vi "Apply Package Name.vi"(8 "error in":errorcluster, 10 "Package Name":string, 11 "gRPC Message Metadata in":T1[](array[typedef])) -> (0 "error out":errorcluster, 3 "gRPC Message Metadata":T1[](array[typedef]))   [LabVIEW 2019, in "grpc-lvsupport.lvlib"]
uses:
  grpc-lvsupport.lvlib
  Message Metadata.ctl
  Message Element Metadata.ctl
  Message Element Type.ctl
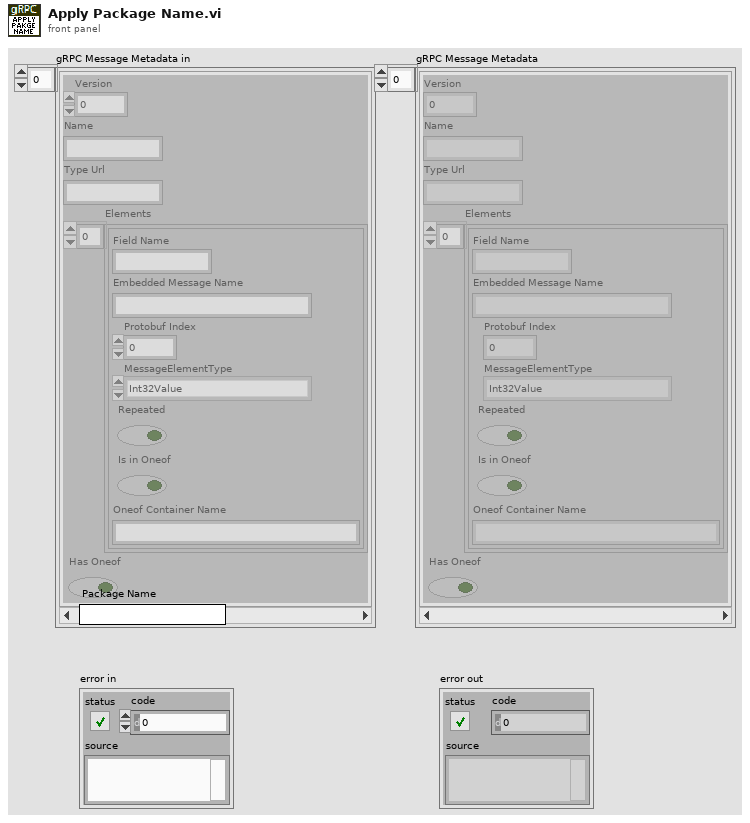
[diagram p1: front panel]
types:
  T1 = typedef "grpc-lvsupport.lvlib/Message Metadata.ctl" = cluster{"Version":i32, "Name":string, "Type Url":string, "Elements":T2[], "Has Oneof":bool}
  T2 = typedef "grpc-lvsupport.lvlib/Message Element Metadata.ctl" = cluster{"Field Name":string, "Embedded Message Name":string, "Protobuf Index":i32, "MessageElementType":T3, "Repeated":bool, "Is in Oneof":bool, "Oneof Container Name":string}
  T3 = typedef "grpc-lvsupport.lvlib/Message Element Type.ctl" = enum32{"Int32Value", "FloatValue", "DoubleValue", "BoolValue", "StringValue", "MessageValue", "Int64Value", "UInt32Value", "UInt64Value", "EnumValue", "Bytes", "Fixed64", "Fixed32", "SFixed64", "SFixed32", "SInt64", "SInt32"}
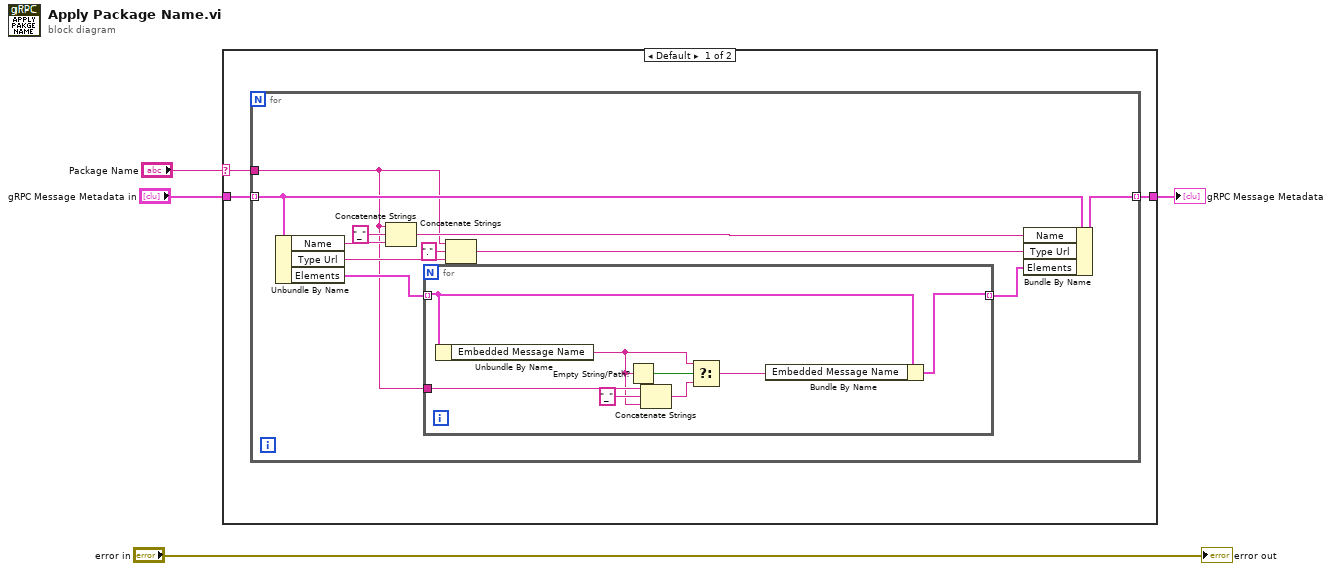
[diagram p0: block diagram]
diagram:
  n1 = case shown="Default" "Package Name" {
    selector: "Package Name" -> [w5 _]
    tunnel: "gRPC Message Metadata in" -> [w7 w27]
    tunnel: [w6 w27] -> w2
    frame Default {
      n2 = for {
        tunnel: w7 -> [w13] mode=indexing
        tunnel: w5 -> [w8]
        tunnel: [w10] -> w6 mode=indexing
        n3 = Unbundle By Name(w13) -> ("Name"=w17:string, "Type Url"=w14:string, "Elements"=w18:T2[])
        n4 = Concatenate Strings(w8, "_" ("string"), w17) -> (w12:string)
        n5 = for {
          tunnel: w18 -> [w23] mode=indexing
          tunnel: [w21] -> w9 mode=indexing
          tunnel: w8 -> [w20]
          n6 = Unbundle By Name(w23) -> ("Embedded Message Name"=w19:string)
          n7 = Empty String/Path?(string/path=w19) -> (empty?=w24:bool)
          n8 = Concatenate Strings(w20, "_" ("string"), w19) -> (w25:string)
          n9 = Select(t=w19, s=w24, f=w25) -> (s? t:f=w22:string)
          n10 = Bundle By Name(cluster=w23, "Embedded Message Name"=w22) -> (w21:T2)
        }
        n11 = Concatenate Strings(w8, "." ("string"), w14) -> (w11:string)
        n12 = Bundle By Name(cluster=w13, "Name"=w12, "Type Url"=w11, "Elements"=w9) -> (w10:T1)
      }
    }
    frame "" {
    }
  }
  "gRPC Message Metadata" <- w2
  "error out" <- "error in"
